vi "TimeSpeedLength_Extractor.vi"(0 "TriggerS1":bool, 7 "TriggerS2":bool, 8 "TriggerS1_prev-1":bool, 9 "TriggerS2_prev-1":bool, 10 "Start_T1_prev":u32, 11 "Start_T2_prev":u32, 12 "Stop_T1_prev":u32, 13 "Flag_RiseEdge_S1_prev":bool) -> (14 "Stop_T1":u32, 15 "Flag_RiseEdge_S1":bool, 16 "Start_T1":u32, 17 "Start_T2":u32, 18 "TriggerS1_prev0":bool, 19 "TriggerS2_prev0":bool, 20 "Length   [mm]":dbl, 22 "Speed [m/s]":dbl, 27 "Stuck_Alarm":bool caption="Time has Elapsed")   [LabVIEW 2020]
panel:
  in  "Time Target (s)":dbl=5.0
  in  "Sensors_Distance [mm]":u32=101
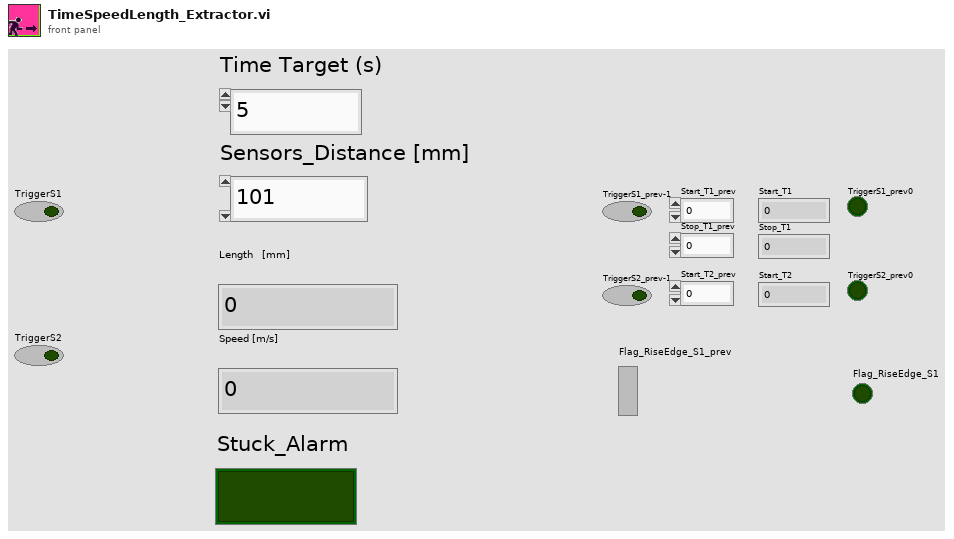
[diagram p1: front panel]
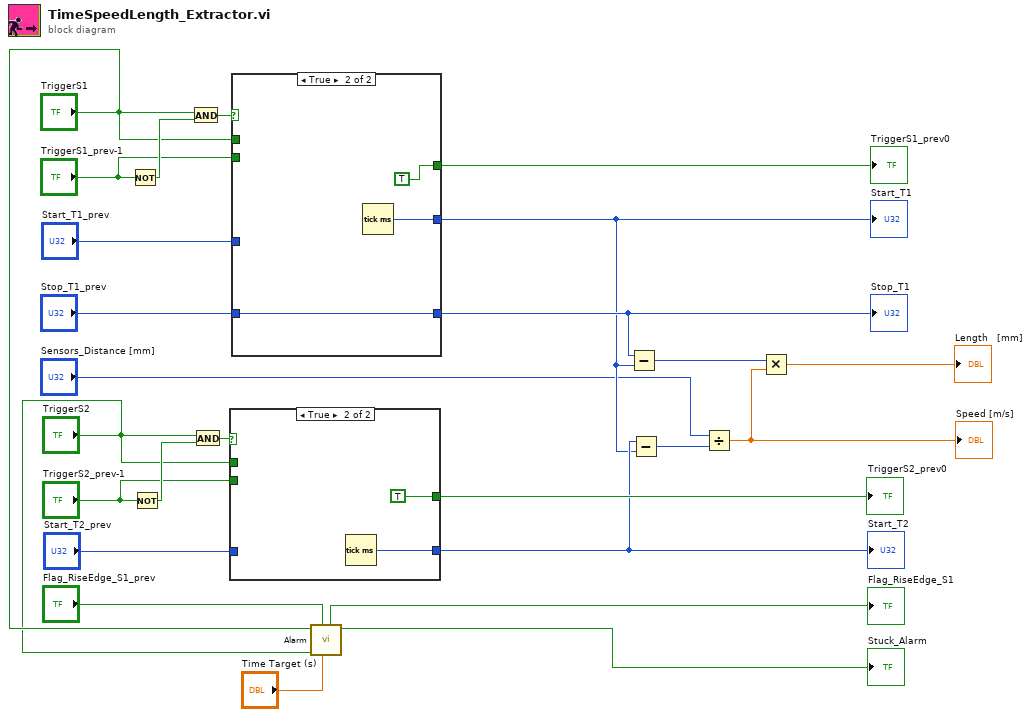
[diagram p0: block diagram]
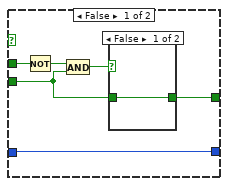
[diagram p2: hidden frame]
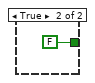
[diagram p3: hidden frame]
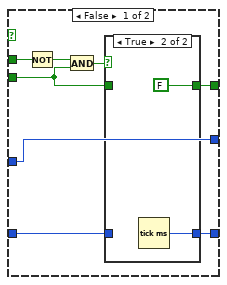
[diagram p4: hidden frame]
diagram:
  n1 = Not(x="TriggerS1_prev-1") -> (.not. x?=w25:bool)
  n2 = Not(x="TriggerS2_prev-1") -> (.not. x?=w19:bool)
  n3 = And(x="TriggerS1", y=w25) -> (x .and. y?=w24:bool)
  n4 = And(x="TriggerS2", y=w19) -> (x .and. y?=w18:bool)
  n5 = case shown="True" w18 {
    tunnel: "TriggerS2" -> [w31 _]
    tunnel: "TriggerS2_prev-1" -> [w27 _]
    tunnel: [w28 TRUE] -> w16
    tunnel: [w26 w34] -> w13
    tunnel: "Start_T2_prev" -> [w26 _]
    frame False {
      n6 = Not(x=w31) -> (.not. x?=w30:bool)
      n7 = And(x=w30, y=w27) -> (x .and. y?=w29:bool)
      n8 = case shown="False" w29 {
        tunnel: [w32 FALSE] -> w28
        tunnel: w27 -> [w32 _]
        frame False {
        }
        frame True {
        }
      }
    }
    frame True {
      n9 = Tick Count (ms)() -> (millisecond timer value=w34:u32)
    }
  }
  "TriggerS2_prev0" <- w16
  "Start_T2" <- w13
  n10 = case shown="True" w24 {
    tunnel: [w43 w50] -> w12
    tunnel: [w38 TRUE] -> w22
    tunnel: "Start_T1_prev" -> [w43 _]
    tunnel: "Stop_T1_prev" -> [w36 w48]
    tunnel: [w39 w48] -> w14
    tunnel: "TriggerS1" -> [w42 _]
    tunnel: "TriggerS1_prev-1" -> [w37 _]
    frame False {
      n11 = Not(x=w42) -> (.not. x?=w41:bool)
      n12 = And(x=w41, y=w37) -> (x .and. y?=w40:bool)
      n13 = case shown="True" w40 {
        tunnel: [w44 w47] -> w39
        tunnel: [w45 FALSE] -> w38
        tunnel: w37 -> [w45 _]
        tunnel: w36 -> [w44 _]
        frame False {
        }
        frame True {
          n14 = Tick Count (ms)() -> (millisecond timer value=w47:u32)
        }
      }
    }
    frame True {
      n15 = Tick Count (ms)() -> (millisecond timer value=w50:u32)
    }
  }
  "Start_T1" <- w12
  "TriggerS1_prev0" <- w22
  "Stop_T1" <- w14
  n16 = call "Alarm.vi"("Time Target (s)"="Time Target (s)", "Flag_RiseEdge_S1_prev"="Flag_RiseEdge_S1_prev", "Trigger_S2"="TriggerS2", "Trigger_S1"="TriggerS1") -> ("Time has Elapsed"=→"Stuck_Alarm":bool, "Flag_RiseEdge_S1"=→"Flag_RiseEdge_S1":bool)  [unwired: 5 in, 1 out]
  n17 = Subtract(x=w14, y=w12) -> (x-y=w9:u32)
  n18 = Subtract(x=w13, y=w12) -> (x-y=w11:u32)
  n19 = Divide(x="Sensors_Distance [mm]", y=w11) -> (x/y=w8:dbl)
  "Speed [m/s]" <- w8
  n20 = Multiply(x=w9, y=w8) -> (x*y=→"Length   [mm]":dbl)
